vi "Close.vi"(8 "error in (no error)":errorcluster, 11 "reference in":refnum<class "Frequency_Counter_Base.lvclass">) -> (0 "error out":errorcluster, 3 "reference in":refnum<class "Frequency_Counter_Base.lvclass">)   [LabVIEW 2022 SP3, in "Frequency_Counter_Base.lvlib" / "Frequency_Counter_Base.lvclass"]
uses:
  Frequency_Counter_Base.lvclass
  Components/ViPER.lvlibp/ViPER.lvclass
  C:/Projects/Medulla/ViPER/Examples/Flux_Capacitor_Tester/Components/ViPER.lvlibp/ViPER.lvclass
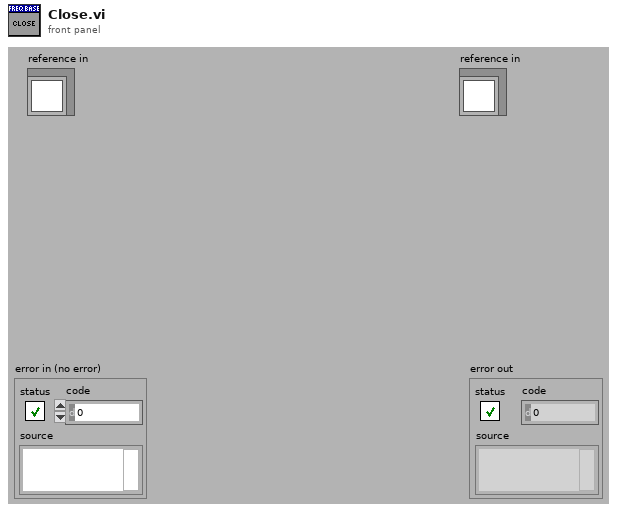
[diagram p1: front panel]
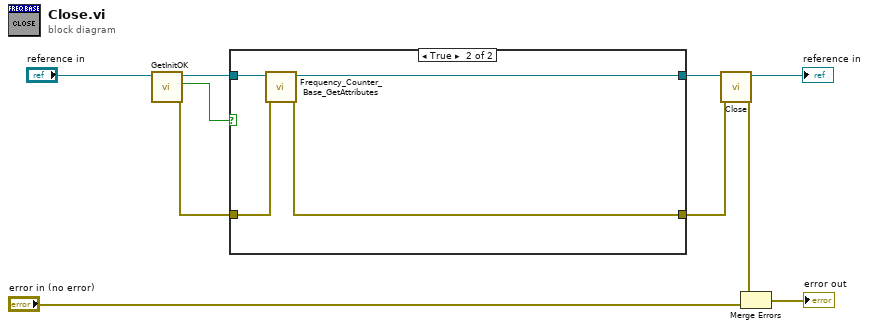
[diagram p0: block diagram]
diagram:
  n1 = call "GetInitOK.vi"("reference in"="reference in") -> ("error out"=w4:errorcluster, "init_ok"=w5:bool, "reference out"=w6:refnum<class "Frequency_Counter_Base.lvclass">)  [unwired: 8 in]
  n2 = case shown="True" w5 {
    tunnel: w4 -> [w12 w15]
    tunnel: [w12 w13] -> w7
    tunnel: w6 -> [w11 w16]
    tunnel: [w11 w14] -> w8
    frame False {
    }
    frame True {
      n3 = call "Frequency_Counter_Base_GetAttributes.vi"("error in (no error)"=w15, "reference in"=w16) -> ("error out"=w13:errorcluster, "reference out"=w14:refnum<class "Frequency_Counter_Base.lvclass">)  [unwired: 6 in, 2 out]
    }
  }
  n4 = call-parent "Close.vi"("error in (no error)"=w7, "reference in"=w8) -> ("error out"=w3:errorcluster, "reference out"=→"reference in":refnum<class "Frequency_Counter_Base.lvclass">)  [unwired: 8 in]
  n5 = Merge Errors(w3, "error in (no error)") -> (→"error out":errorcluster)
